vi "Save_Various_Calculated_Vals_1.vi"(4 "[IN] Save Tracks in Columns":bool, 5 "[IN] Save Mean Vels for Tracks":bool, 6 "[IN] Save Track Durations":bool, 7 "[IN] Save All Path Velocities":bool, 8 "error IN":errorcluster, 9 "[IN] Statistics":T1, 10 "[IN] Save All Instant Velocities":bool, 11 "[IN] File Path with Movie":path) -> (0 "error OUT":errorcluster)   [LabVIEW 2013]
doc: "This subprogram saves all values calculated during the tracking step"
uses:
  <vilib>/Utility/file.llb/Write To Spreadsheet File (DBL).vi
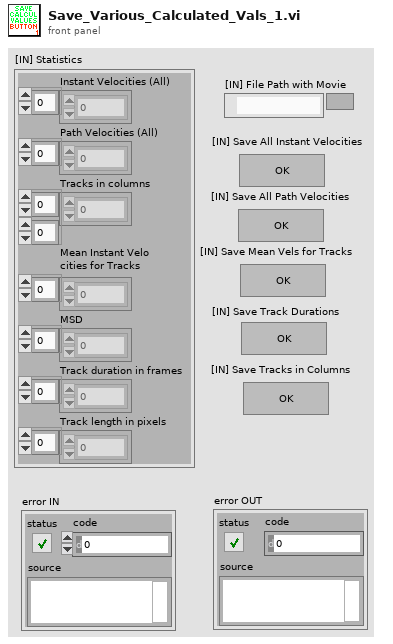
[diagram p1: front panel]
types:
  T1 = cluster{"Instant Velocities (All)":dbl[], "Path Velocities (All) ":dbl[], "Tracks in columns":dbl[][], "Mean Instant Velo\ncities for Tracks":dbl[], "MSD":dbl[], "Track duration in frames":u16[], "Track length in pixels":dbl[]}
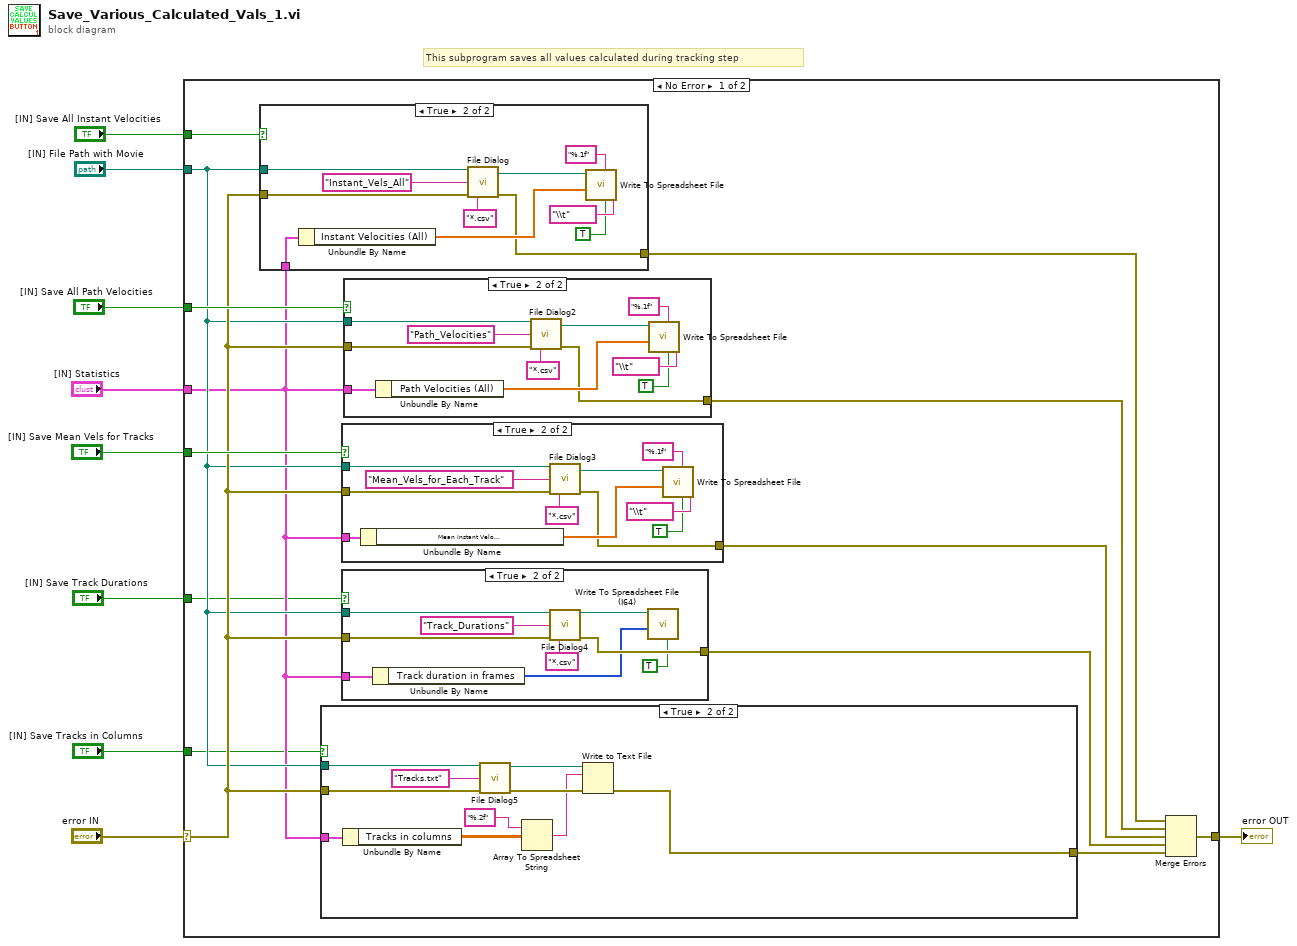
[diagram p0: block diagram]
diagram:
  # "This subprogram saves all values calculated during tracking step"
  n1 = case shown="No Error" "error IN" {
    selector: "error IN" -> [w20 w81]
    tunnel: "[IN] File Path with Movie" -> [w19 _]
    tunnel: [w16 w81] -> w7
    tunnel: "[IN] Save All Instant Velocities" -> [w23 _]
    tunnel: "[IN] Statistics" -> [w18 _]
    tunnel: "[IN] Save All Path Velocities" -> [w22 _]
    tunnel: "[IN] Save Mean Vels for Tracks" -> [w21 _]
    tunnel: "[IN] Save Tracks in Columns" -> [w17 _]
    tunnel: "[IN] Save Track Durations" -> [w11 _]
    frame No Error {
      n2 = case shown="True" w23 {
        tunnel: w19 -> [_ w75]
        tunnel: w20 -> [w69 w73]
        tunnel: w18 -> [_ w72]
        tunnel: [w69 w70] -> w12
        frame False {
        }
        frame True {
          n3 = Unbundle By Name(w72) -> ("Instant Velocities (All)"=w71:dbl[])
          n4 = call "File Dialog"("start path"=w75, "default name"="Instant_Vels_All", "error in"=w73, "pattern (all files)"="*.csv") -> ("selected path"=w77:path, "error out"=w70:errorcluster)  [unwired: 8 in, 2 out]
          n5 = call-poly <vilib>:"Write To Spreadsheet File.vi"("delimiter (\\t)"="\\t" ("delimiter (\\t)"), "transpose? (no:F)"=TRUE, "format (%.3f)"="%.1f", "1D data"=w71, "file path (dialog if empty)"=w77) -> ()  [unwired: 3 in, 1 out]
        }
      }
      n6 = case shown="True" w17 {
        tunnel: w19 -> [_ w33]
        tunnel: w20 -> [w24 w32]
        tunnel: w18 -> [_ w34]
        tunnel: [w24 w26] -> w10
        frame False {
        }
        frame True {
          n7 = Unbundle By Name(w34) -> ("Tracks in columns"=w30:dbl[][])
          n8 = call "File Dialog5"("start path"=w33, "default name"="Tracks.txt", "error in"=w32) -> ("selected path"=w28:path, "error out"=w29:errorcluster)  [unwired: 9 in, 2 out]
          n9 = Array To Spreadsheet String(array=w30, 3:"%.2f" ("format string")) -> (spreadsheet string=w27:string)  [unwired: 1 in]
          n10 = Write to Text File(file (use dialog)=w28, text=w27, error in=w29) -> (error out=w26:errorcluster)  [unwired: 1 in, 2 out]
        }
      }
      n11 = case shown="True" w21 {
        tunnel: w19 -> [_ w51]
        tunnel: w20 -> [w45 w49]
        tunnel: w18 -> [_ w48]
        tunnel: [w45 w46] -> w14
        frame False {
        }
        frame True {
          n12 = Unbundle By Name(w48) -> ("Mean Instant Velo\ncities for Tracks"=w47:dbl[])
          n13 = call "File Dialog3"("start path"=w51, "default name"="Mean_Vels_for_Each_Track", "error in"=w49, "pattern (all files)"="*.csv") -> ("selected path"=w53:path, "error out"=w46:errorcluster)  [unwired: 8 in, 2 out]
          n14 = call-poly <vilib>:"Write To Spreadsheet File.vi"("delimiter (\\t)"="\\t" ("delimiter (\\t)"), "transpose? (no:F)"=TRUE, "format (%.3f)"="%.1f", "1D data"=w47, "file path (dialog if empty)"=w53) -> ()  [unwired: 3 in, 1 out]
        }
      }
      n15 = case shown="True" w11 {
        tunnel: w19 -> [_ w43]
        tunnel: w20 -> [w35 w41]
        tunnel: w18 -> [_ w40]
        tunnel: [w35 w39] -> w15
        frame False {
        }
        frame True {
          n16 = Unbundle By Name(w40) -> ("Track duration in frames"=w36:u16[])
          n17 = call "File Dialog4"("start path"=w43, "default name"="Track_Durations", "error in"=w41, "pattern (all files)"="*.csv") -> ("selected path"=w38:path, "error out"=w39:errorcluster)  [unwired: 8 in, 2 out]
          n18 = call <vilib>:"Write To Spreadsheet File (I64).vi"("transpose? (no:F)"=TRUE, "1D data"=w36, "file path (dialog if empty)"=w38) -> ()  [unwired: 5 in, 1 out]
        }
      }
      n19 = case shown="True" w22 {
        tunnel: w19 -> [_ w63]
        tunnel: w20 -> [w57 w61]
        tunnel: w18 -> [_ w60]
        tunnel: [w57 w58] -> w13
        frame False {
        }
        frame True {
          n20 = Unbundle By Name(w60) -> ("Path Velocities (All)"=w59:dbl[])
          n21 = call "File Dialog2"("start path"=w63, "default name"="Path_Velocities", "error in"=w61, "pattern (all files)"="*.csv") -> ("selected path"=w65:path, "error out"=w58:errorcluster)  [unwired: 8 in, 2 out]
          n22 = call-poly <vilib>:"Write To Spreadsheet File.vi"("delimiter (\\t)"="\\t" ("delimiter (\\t)"), "transpose? (no:F)"=TRUE, "format (%.3f)"="%.1f", "1D data"=w59, "file path (dialog if empty)"=w65) -> ()  [unwired: 3 in, 1 out]
        }
      }
      n23 = Merge Errors(w12, w13, w14, w15, w10) -> (w16:errorcluster)
    }
    frame Error {
    }
  }
  "error OUT" <- w7
